vi "Read All-Ctrl-Data.vi"(8 "error in (no error)":errorcluster, 11 "Quick-GUI-Update in":refnum<class "Quick-GUI-Update.lvclass">) -> (0 "error out":errorcluster, 2 "All-Ctrl-Data":T1(c390), 3 "Quick-GUI-Update out":refnum<class "Quick-GUI-Update.lvclass">)   [LabVIEW 2020, in "Easy GUI Operation.lvlib" / "Quick-GUI-Update.lvclass"]
uses:
  Quick-GUI-Update.lvclass
  Quick-GUI-Update.lvclass/Quick-GUI-Update.ctl
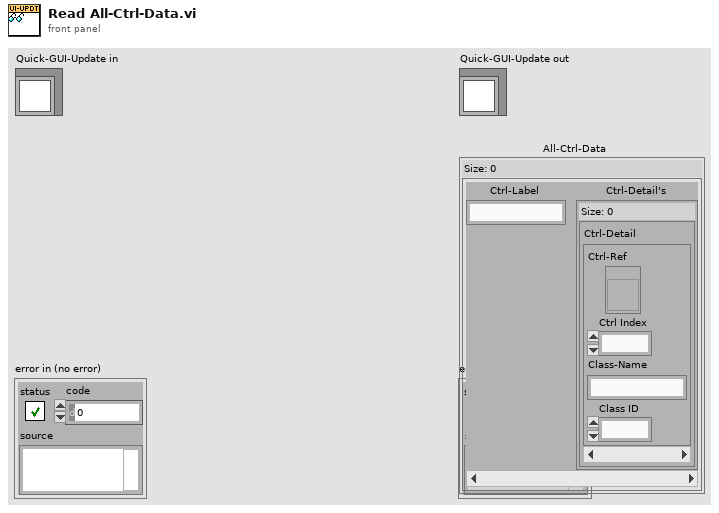
[diagram p1: front panel]
types:
  T1 = map{string, set{cluster{"Ctrl-Ref":refnum<vi>, "Ctrl Index":i32, "Class-Name":string, "Class ID":u32}}}
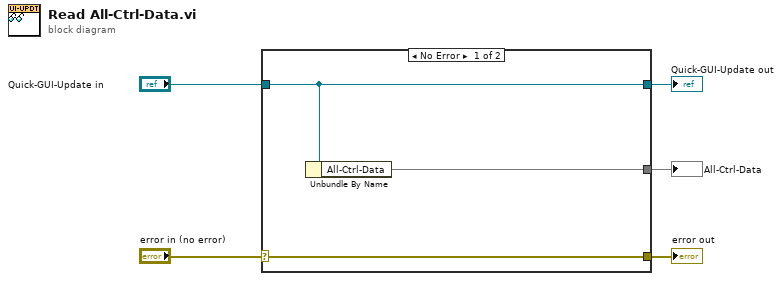
[diagram p0: block diagram]
diagram:
  n1 = case shown="No Error" "error in (no error)" {
    selector: "error in (no error)" -> [w8 w9]
    tunnel: [w8 w9] -> w4
    tunnel: [w7 w10] -> w2
    tunnel: "Quick-GUI-Update in" -> [w7 w10]
    tunnel: [w6 _] -> w1
    frame No Error {
      n2 = Unbundle By Name(w7) -> ("All-Ctrl-Data"=w6:T1)
    }
    frame Error {
    }
  }
  "error out" <- w4
  "Quick-GUI-Update out" <- w2
  "All-Ctrl-Data" <- w1
